vi "SSC DAQmx Configure Digital Edge Start trigger.vi"(0 "DAQmx SSC in":T1[](array[typedef]), 5 "Source":tag, 7 "Edge":i32(ring)=10280 items=["Rising"=10280, "Falling"=10171], 11 "error in":errorcluster) -> (4 "DAQmx SSC out":T1[](array[typedef]), 15 "error out":errorcluster)   [LabVIEW 2020]
doc: "Configures the task to start acquiring or generating samples on a rising or falling edge of a digital signal."
uses:
  Pin Map/SSC DAQmx.ctl
  <vilib>/DAQmx/configure/trigger.llb/DAQmx Start Trigger (Digital Edge).vi
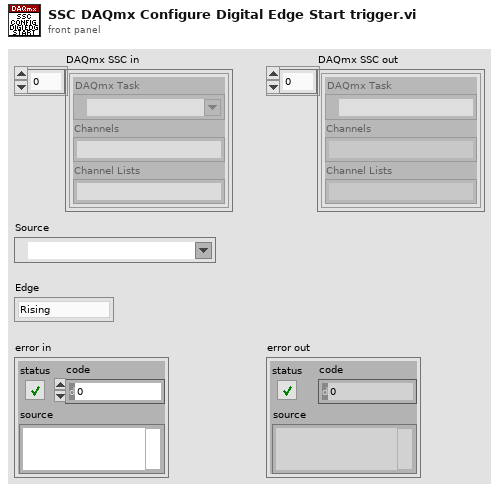
[diagram p1: front panel]
types:
  T1 = typedef "SSC DAQmx.ctl" = cluster{"DAQmx Task ":refnum<k21>, "Channels":string, "Channel Lists":string}
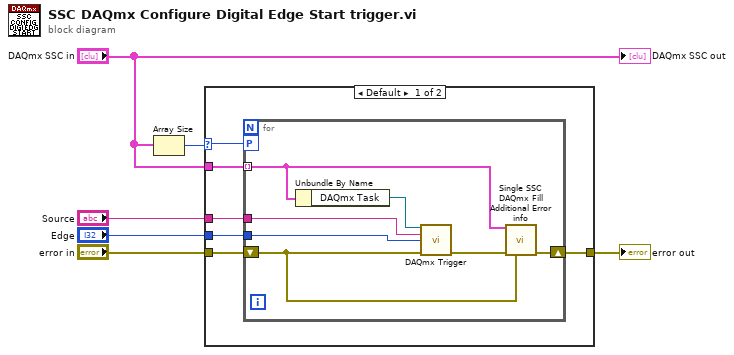
[diagram p0: block diagram]
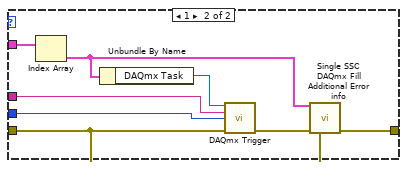
[diagram p2: hidden frame]
diagram:
  n1 = Array Size(array="DAQmx SSC in") -> (size(s)=w4:i32)
  n2 = case shown="Default" w4 {
    selector: w4 -> [w10 _]
    tunnel: [w12 w27] -> w6
    tunnel: "error in" -> [w11 w26]
    tunnel: "DAQmx SSC in" -> [w9 w25]
    tunnel: "Edge" -> [w8 w24]
    tunnel: "Source" -> [w7 w23]
    frame Default {
      n3 = for {
        tunnel: w9 -> [w18] mode=indexing
        workers-P: w10 -> [_]
        shift-right: [w19] -> w12
        shift-left: w11 -> [w17]
        tunnel: w8 -> [w14]
        tunnel: w7 -> [w13]
        n4 = Unbundle By Name(w18) -> ("DAQmx Task"=w15:refnum<k21>)
        n5 = call-poly <vilib>:"DAQmx Trigger.vi"("task/channels in"=w15, "source"=w13, "edge"=w14, "error in"=w17) -> ("error out"=w16:errorcluster)  [unwired: 10 in, 1 out]
        n6 = call "Single SSC DAQmx Fill Additional Error info.vi"("DAQmx SSC in"=w18, "error in"=w16, "previous error in"=w17) -> ("error out"=w19:errorcluster)  [unwired: 12 in]
      }
    }
    frame 1 {
      n7 = Index Array(array=w25) -> (element=w20:T1)  [unwired: 1 in]
      n8 = Unbundle By Name(w20) -> ("DAQmx Task"=w21:refnum<k21>)
      n9 = call-poly <vilib>:"DAQmx Trigger.vi"("task/channels in"=w21, "source"=w23, "edge"=w24, "error in"=w26) -> ("error out"=w22:errorcluster)  [unwired: 10 in, 1 out]
      n10 = call "Single SSC DAQmx Fill Additional Error info.vi"("DAQmx SSC in"=w20, "error in"=w22, "previous error in"=w26) -> ("error out"=w27:errorcluster)  [unwired: 12 in]
    }
  }
  "error out" <- w6
  "DAQmx SSC out" <- "DAQmx SSC in"
